vi "Save DG measurement.vi"(6 "Index":i32, 7 "DG measurement":T1={"Signal frequencies (Hz)"=[1000.0], "Signal amplitudes (V)"=[0.707], "Sampling frequencies (Hz)"=[10000000.0], "Record lengths (multiples of periods)"=[10000.0], "Calculate results"=FALSE, "Algorithm"="TWM-PJVSSubS", "TWM data directories"=[], "TWM data directories relative"=[], "PJVS frequencies (Hz)"=[1000.0], "PJVS reference voltages array of vector cluster"=[], "Requested PJVS steps"=[20], "Data folder"=path "", "Rs"=0, "Re"=0, "Settle down after PJVS change (s)"=1.0, "Switch position"=0.0, "PJVS amplitudes (Hz)"=[1000.0], "DG measurement info files"=[]} {"PJVS amplitudes (Hz)" format="%#_3p"; "PJVS reference voltages array of vector cluster"."PJVS reference voltages vector" format="%#_3p"; "PJVS frequencies (Hz)" format="%#_3p"; "Record lengths (multiples of periods)" format="%#_3p"; "Sampling frequencies (Hz)" format="%#_3p"; "Signal amplitudes (V)" format="%#_3p"; "Signal frequencies (Hz)" format="%#_3p"}, 8 "error in":errorcluster, 9 "Set PJVS steps":u32) -> (0 "error out":errorcluster)   [LabVIEW 2020]
doc: "Save SS measurement informations into info file."
uses:
  DG Measurement/DG measurement.ctl
  external libraries/TWM-1.8.7.0-client/EXT.vi
  external libraries/TWM-1.8.7.0-client/String.vi
  external libraries/TWM-1.8.7.0-client/I64.vi
  external libraries/TWM-1.8.7.0-client/1D EXT.vi
  external libraries/TWM-1.8.7.0-client/U64.vi
  external libraries/TWM-1.8.7.0-client/infolib.lvlib
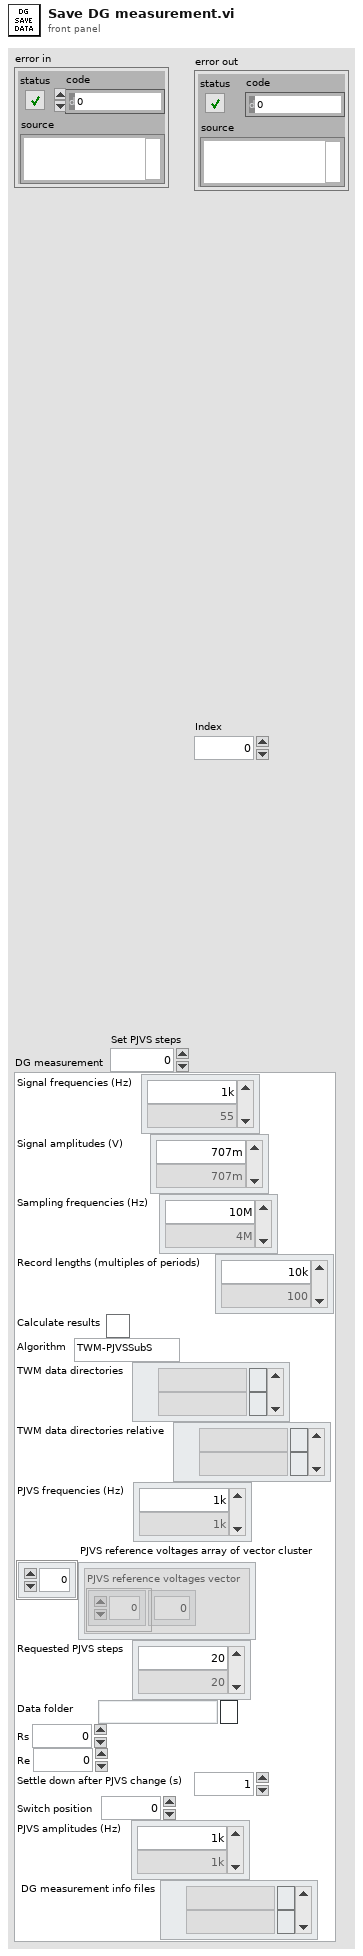
[diagram p1: front panel]
types:
  T1 = typedef "DG measurement.ctl" = cluster{"Signal frequencies (Hz)":dbl[], "Signal amplitudes (V)":dbl[], "Sampling frequencies (Hz)":dbl[], "Record lengths (multiples of periods)":dbl[], "Calculate results":bool, "Algorithm":string, "TWM data directories":path[], "TWM data directories relative":path[], "PJVS frequencies (Hz)":dbl[], "PJVS reference voltages array of vector cluster":cluster{"PJVS reference voltages vector":dbl[]}[], "Requested PJVS steps":u32[], "Data folder":path, "Rs":i32, "Re":i32, "Settle down after PJVS change (s)":dbl, "Switch position":dbl, "PJVS amplitudes (Hz)":dbl[], "DG measurement info files":path[]}
  T2 = cluster{"PJVS reference voltages vector":dbl[]}[]
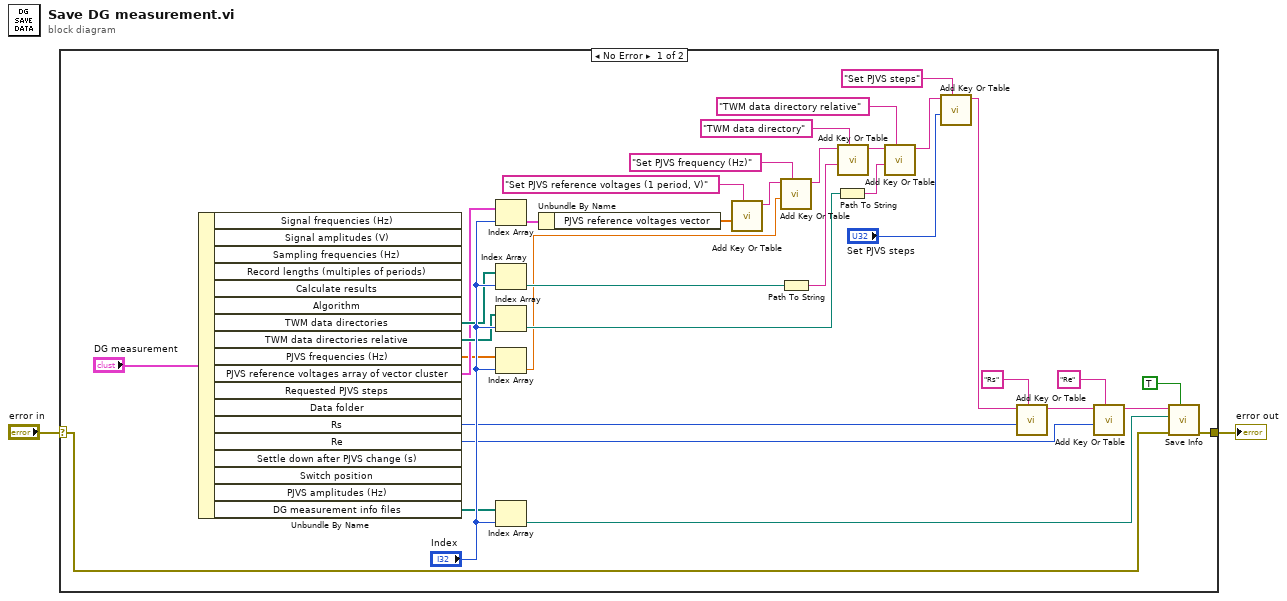
[diagram p0: block diagram]
diagram:
  n1 = case shown="No Error" "error in" {
    selector: "error in" -> [w28 w38]
    tunnel: [w29 w38] -> w2
    frame No Error {
      n2 = Unbundle By Name("DG measurement") -> ("TWM data directories"=w6:path[], "TWM data directories relative"=w7:path[], "PJVS frequencies (Hz)"=w4:dbl[], "PJVS reference voltages array of vector cluster"=w5:T2, "Rs"=w10:i32, "Re"=w9:i32, "DG measurement info files"=w8:path[])  [unwired: 11 out]
      n3 = Index Array(array=w5, index="Index") -> (element=w13:cluster{"PJVS reference voltages vector":dbl[]})
      n4 = Index Array(array=w6, index="Index") -> (element=w20:path)
      n5 = Index Array(array=w7, index="Index") -> (element=w18:path)
      n6 = Index Array(array=w4, index="Index") -> (element=w15:dbl)
      n7 = Index Array(array=w8, index="Index") -> (element=w16:path)
      n8 = Unbundle By Name(w13) -> ("PJVS reference voltages vector"=w12:dbl[])
      n9 = call-poly "Add Key Or Table.vi"("key description"="Set PJVS reference voltages (1 period, V)", "numeric"=w12) -> ("info data out"=w34:string)  [unwired: 8 in, 1 out]
      n10 = call-poly "Add Key Or Table.vi"("key description"="Set PJVS frequency (Hz)", "numeric"=w15, "info data"=w34) -> ("info data out"=w33:string)  [unwired: 7 in, 1 out]
      n11 = Path To String(path=w20) -> (string=w19:string)
      n12 = Path To String(path=w18) -> (string=w17:string)
      n13 = call-poly "Add Key Or Table.vi"("key description"="TWM data directory", "string"=w19, "info data"=w33) -> ("info data out"=w27:string)  [unwired: 7 in, 1 out]
      n14 = call-poly "Add Key Or Table.vi"("key description"="TWM data directory relative", "string"=w17, "info data"=w27) -> ("info data out"=w26:string)  [unwired: 7 in, 1 out]
      n15 = call-poly "Add Key Or Table.vi"("key description"="Set PJVS steps", "numeric"="Set PJVS steps", "info data"=w26) -> ("info data out"=w3:string)  [unwired: 7 in, 1 out]
      n16 = call-poly "Add Key Or Table.vi"("key description"="Rs", "numeric"=w10, "info data"=w3) -> ("info data out"=w22:string)  [unwired: 7 in, 1 out]
      n17 = call-poly "Add Key Or Table.vi"("key description"="Re", "numeric"=w9, "info data"=w22) -> ("info data out"=w21:string)  [unwired: 7 in, 1 out]
      n18 = call "Save Info.vi"("Overwrite? (T)"=TRUE, "error in"=w28, "filename"=w16, "info data"=w21) -> ("error out"=w29:errorcluster)  [unwired: 7 in]
    }
    frame Error {
    }
  }
  "error out" <- w2
